vi "Lesson5 - bundles.vi"() -> ()   [LabVIEW 2013]
panel:
  out "String 2":string
  out "String":string
  out "Cluster 2":T1
  in  "Cluster":T2
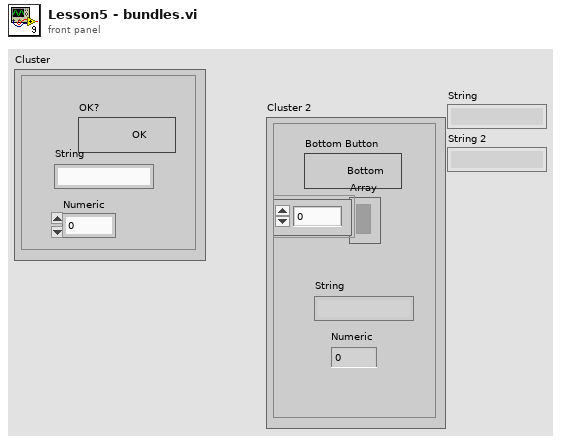
[diagram p1: front panel]
types:
  T1 = cluster{"Bottom Button":bool, "Array":bool[], "String":string, "Numeric":dbl}
  T2 = cluster{"OK?":bool, "String":string, "Numeric":dbl}
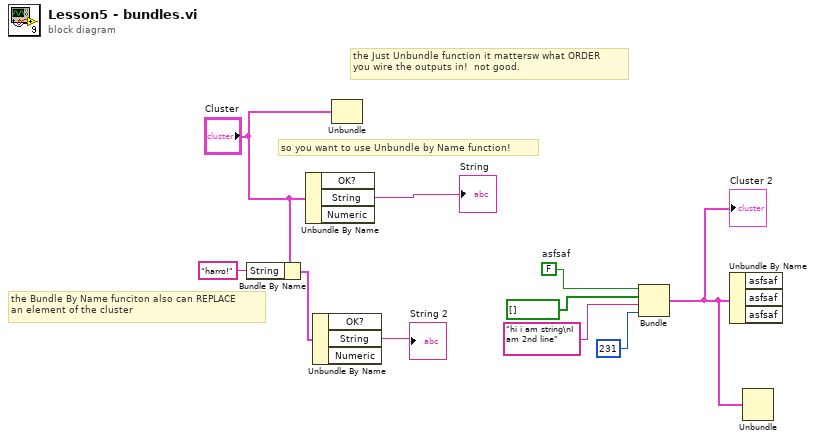
[diagram p0: block diagram]
diagram:
  w9 = FALSE  # asfsaf
  # "the Bundle By Name funciton also can REPLACE\nan element of the cluster"
  # "so you want to use Unbundle by Name function!"
  # "the Just Unbundle function it mattersw what ORDER\nyou wire the outputs in!  not good."
  n1 = Bundle By Name "Bundle By Name"(cluster="Cluster", "String"="harro!") -> (w1:T2)
  n2 = Unbundle By Name "Unbundle By Name"("Cluster") -> ("String"=→"String":string)  [unwired: 2 out]
  n3 = Unbundle By Name "Unbundle By Name"(w1) -> ("String"=→"String 2":string)  [unwired: 2 out]
  n4 = Unbundle "Unbundle"("Cluster") -> ()  [unwired: 3 out]
  n5 = Bundle "Bundle"("asfsaf"=w9, bool[] [], "hi i am string\nI am 2nd line", 231) -> (w6:cluster{"asfsaf":bool, bool[], string, i32})  [unwired: 1 in]
  "Cluster 2" <- w6
  n6 = Unbundle By Name "Unbundle By Name"(w6) -> ()  [unwired: 3 out]
  n7 = Unbundle(w6) -> ()  [unwired: 4 out]
